vi "InitBorder.vi"(1 "引用簇":T1, 2 "error in (no error)":errorcluster caption="错误输入（无错误）") -> (0 "error in (no error) 2":errorcluster caption="错误输出（无错误）")   [LabVIEW 2012]
uses:
  <vilib>/Utility/miscctls.llb/LVBoundsTypeDef.ctl
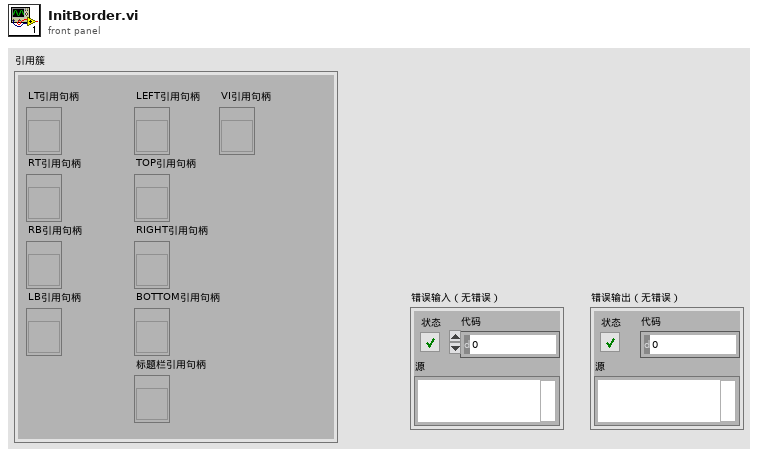
[diagram p1: front panel]
types:
  T1 = cluster{"LEFT引用句柄":refnum<vi>, "TOP引用句柄":refnum<vi>, "RIGHT引用句柄":refnum<vi>, "BOTTOM引用句柄":refnum<vi>, "VI引用句柄":refnum<vi>, "标题栏引用句柄 ":refnum<vi>, "LT引用句柄":refnum<vi>, "RT引用句柄":refnum<vi>, "RB引用句柄":refnum<vi>, "LB引用句柄":refnum<vi>}
  T2 = typedef "LVBoundsTypeDef.ctl" = cluster{"Width":u32, "Height":u32}
  T3 = typedef "LVRectTypeDef.ctl" = cluster{"Left":i16, "Top":i16, "Right":i16, "Bottom":i16}
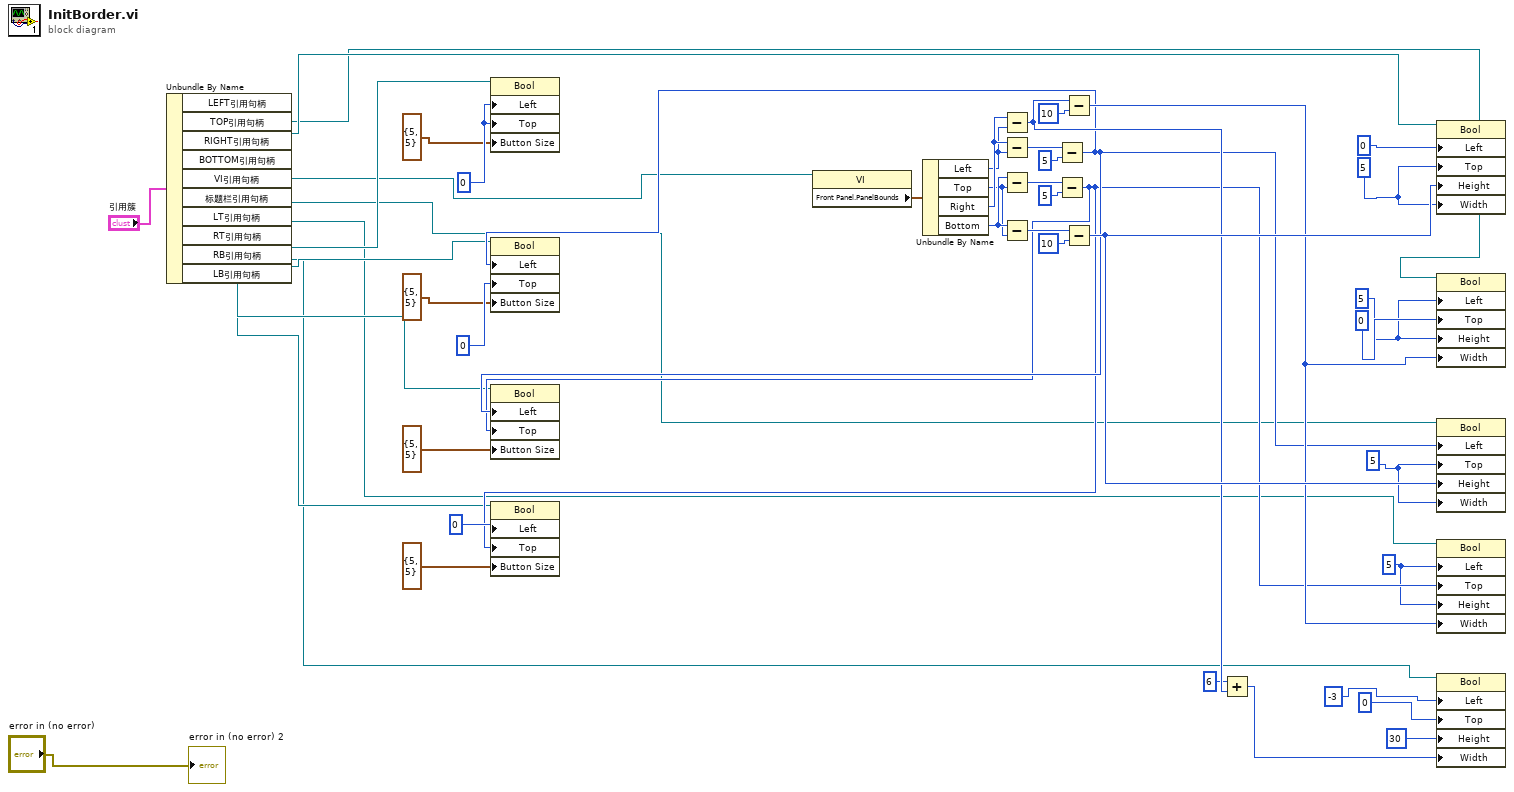
[diagram p0: block diagram]
diagram:
  w28 = 0
  w20 = 5 ("位置:置顶")
  w18 = 5 ("位置:置顶")
  w17 = 5 ("位置:置顶")
  w19 = 5 ("位置:置顶")
  n1 = Unbundle By Name("引用簇") -> ("LEFT引用句柄"=w5:refnum<vi>, "TOP引用句柄"=w4:refnum<vi>, "RIGHT引用句柄"=w3:refnum<vi>, "BOTTOM引用句柄"=w2:refnum<vi>, "VI引用句柄"=w6:refnum<vi>, "标题栏引用句柄"=w1:refnum<vi>, "LT引用句柄"=w10:refnum<vi>, "RT引用句柄"=w9:refnum<vi>, "RB引用句柄"=w8:refnum<vi>, "LB引用句柄"=w7:refnum<vi>)
  n2 = property class="Bool"(reference=w10, "Left"=w28, "Top"=w28, "Button Size"=T2 {"Width"=5, "Height"=5} ("按钮大小")) -> ()  [unwired: 1 in, 2 out]
  n3 = property class="VI"(reference=w6) -> ("Front Panel.PanelBounds"=w45:T3)  [unwired: 1 in, 2 out]
  n4 = Unbundle By Name(w45) -> ("Left"=w39:i16, "Top"=w33:i16, "Right"=w40:i16, "Bottom"=w34:i16)
  n5 = Subtract(x=w40, y=w39) -> (x-y=w29:i16)
  n6 = Subtract(x=w40, y=w39) -> (x-y=w38:i16)
  n7 = Subtract(x=w34, y=w33) -> (x-y=w35:i16)
  n8 = Subtract(x=w34, y=w33) -> (x-y=w44:i16)
  n9 = Subtract(x=w38, y=5 ("位置:居左")) -> (x-y=w25:i32)
  n10 = property class="Bool"(reference=w9, "Left"=w25, "Top"=0 ("位置:置顶"), "Button Size"=T2 {"Width"=5, "Height"=5} ("按钮大小")) -> ()  [unwired: 1 in, 2 out]
  n11 = Subtract(x=w35, y=5 ("位置:居左")) -> (x-y=w24:i32)
  n12 = property class="Bool"(reference=w8, "Left"=w25, "Top"=w24, "Button Size"=T2 {"Width"=5, "Height"=5} ("按钮大小")) -> ()  [unwired: 1 in, 2 out]
  n13 = property class="Bool"(reference=w7, "Left"=0 ("位置:居左"), "Top"=w24, "Button Size"=T2 {"Width"=5, "Height"=5} ("按钮大小")) -> ()  [unwired: 1 in, 2 out]
  n14 = Subtract(x=w29, y=10 ("位置:居左")) -> (x-y=w30:i32)
  n15 = Subtract(x=w44, y=10 ("位置:居左")) -> (x-y=w42:i32)
  n16 = Add(x=6 ("位置:置顶"), y=w29) -> (x+y=w22:i32)
  n17 = property class="Bool"(reference=w5, "Left"=0 ("位置:居左"), "Top"=w20, "Height"=w42, "Width"=w20) -> ()  [unwired: 1 in, 2 out]
  n18 = property class="Bool"(reference=w4, "Left"=w19, "Top"=0 ("位置:置顶"), "Height"=w19, "Width"=w30) -> ()  [unwired: 1 in, 2 out]
  n19 = property class="Bool"(reference=w3, "Left"=w25, "Top"=w18, "Height"=w42, "Width"=w18) -> ()  [unwired: 1 in, 2 out]
  n20 = property class="Bool"(reference=w2, "Left"=w17, "Top"=w24, "Height"=w17, "Width"=w30) -> ()  [unwired: 1 in, 2 out]
  n21 = property class="Bool"(reference=w1, "Left"=-3 ("位置:置顶"), "Top"=0 ("位置:置顶"), "Height"=u32 30 ("按钮大小:高度"), "Width"=w22) -> ()  [unwired: 1 in, 2 out]
  "error in (no error) 2" <- "error in (no error)"
